vi "Get Board Properties.vi"(0 "Communication Bus Template Interfaces:Implementation.lvlib:Shared Resources.lvclass":refnum<class "Shared Resources.lvclass">, 11 "error in":errorcluster) -> (6 "Board ID":i32, 8 "Port Speed":T1 items=["FDX_100MBIT"=0, "FDX_10MBIT"=1, "FDX_1000MBIT"=5, "FDX_AUTO_100MBIT"=2, "FDX_AUTO_10MBIT"=3], 10 "Port Configuration":u32, 15 "error out":errorcluster)   [LabVIEW 2020, in "AIM ARINC 664 Engine.lvlib" / "Implementation.lvlib" / "Shared Resources.lvclass"]
uses:
  Shared Resources.lvclass
  <instrlib>/AIM GmbH/_AIM 664/_controls/port_speed.ctl
  Shared Resources.lvclass/Shared Resources.ctl
  <instrlib>/AIM GmbH/_AIM 664/AIM664LV.lvlib
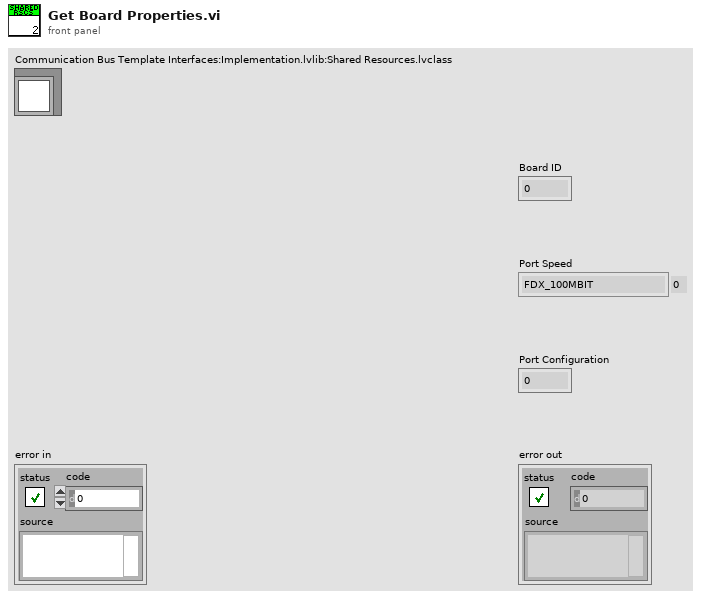
[diagram p1: front panel]
types:
  T1 = typedef "AIM664LV.lvlib/port_speed.ctl" = u32
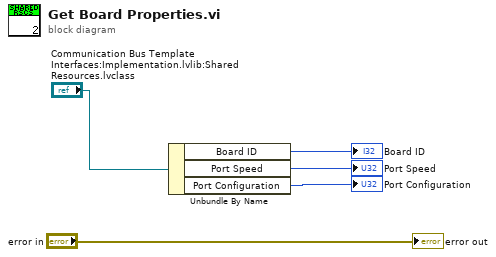
[diagram p0: block diagram]
diagram:
  n1 = Unbundle By Name("Communication Bus Template Interfaces:Implementation.lvlib:Shared Resources.lvclass") -> ("Board ID"=→"Board ID":i32, "Port Speed"=→"Port Speed":T1, "Port Configuration"=→"Port Configuration":u32)
  "error out" <- "error in"
